vi "JSON to LVObject.vi"(7 "Demo LVClass Serializer in":refnum<class "Demo LVClass Serializer.lvclass">, 8 "error in (no error)":errorcluster, 9 "Object Type":refnum<class>, 10 "Offset":i32, 11 "JSON":string) -> (0 "error out":errorcluster, 1 "Object":refnum<class>)   [LabVIEW 2017, in "Demo LVClass Serializer.lvclass"]
uses:
  Demo LVClass Serializer.lvclass
  JSONtext.lvlib
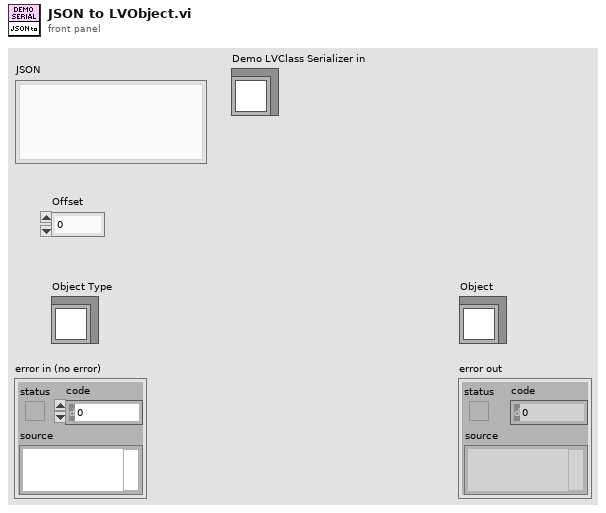
[diagram p1: front panel]
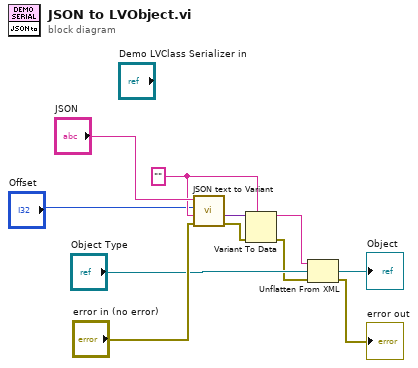
[diagram p0: block diagram]
diagram:
  w9 = ""
  n1 = call "JSON text to Variant.vi"("error in (no error)"="error in (no error)", "Data Type"=w9, "Offset"="Offset", "JSON"="JSON") -> ("error out"=w8:errorcluster, "Variant out"=w10:variant)  [unwired: 6 in]
  n2 = Variant To Data(error in=w8, type=w9, Variant=w10) -> (data=w6:string, error out=w3:errorcluster)
  n3 = Unflatten From XML(xml string=w6, type="Object Type", error in (no error)=w3) -> (value=→"Object":refnum<class>, error out=→"error out":errorcluster)
